vi "Get-client-channels-by-type.vi"(8 "error in (no error)":errorcluster, 10 "Module type":T1, 11 "ModComm in":T2) -> (0 "error out":errorcluster, 2 "Client channels":refnum<queue>[](array[refnum]), 3 "ModComm out":T2)   [LabVIEW 2013, in "Server.lvlib" / "Server.lvclass"]
uses:
  Server.lvclass
  Object-reference.ctl
  Supported-module-types.ctl
  Messages/Sources/Message.lvclass
  Server.lvclass/Server.ctl
  Read Clients.vi
  Read Client channels.vi
  Read Server channel.vi
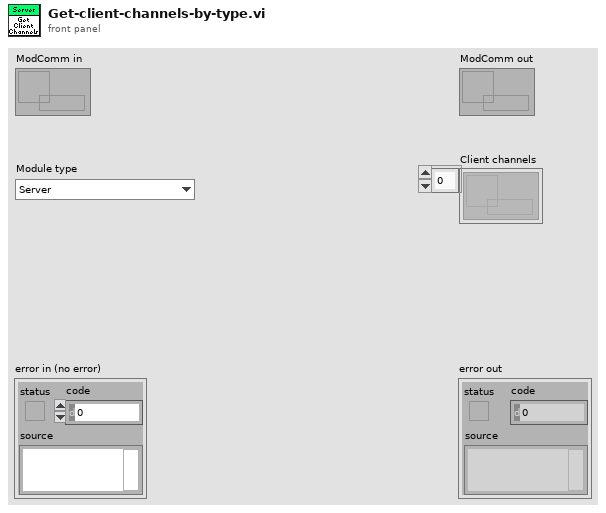
[diagram p1: front panel]
types:
  T1 = typedef "Server.lvlib/Server.lvclass/Supported-module-types.ctl" = enum16{"Server", "All", "BeamControl", "PowderDeposition", "StrategyParser", "CameraVision", "MaterialCharacterization", "StatusMonitor", "SLMSimulation", "LaserCharacterization"}
  T2 = typedef "Server.lvlib/Server.lvclass/Object-reference.ctl" = refnum<data-value>
  T3 = typedef "Module-communication.lvlib/Server.lvclass/Supported-module-types.ctl" = enum16{"Server", "All", "BeamControl", "PowderDeposition", "StrategyParser", "CameraVision", "MaterialCharacterization", "StatusMonitor", "SLMSimulation", "LaserCharacterization"}
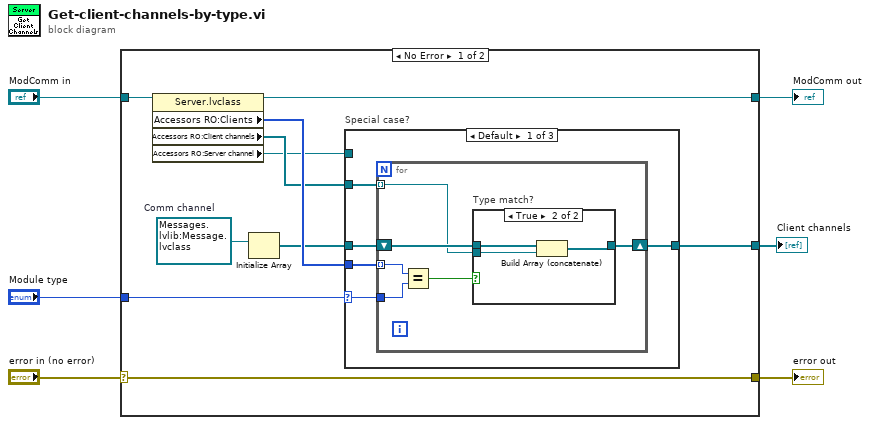
[diagram p0: block diagram]
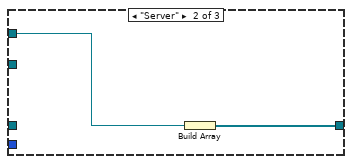
[diagram p3: hidden frame]
diagram:
  n1 = case shown="No Error" "error in (no error)" {
    selector: "error in (no error)" -> [w16 w36]
    tunnel: [w16 w36] -> w5
    tunnel: [w14 w35] -> w3
    tunnel: "ModComm in" -> [w15 w35]
    tunnel: "Module type" -> [w7 _]
    tunnel: [w12 _] -> w1
    frame No Error {
      w10 = refnum<queue> refnum  # Comm channel
      n2 = property class="Server.lvclass"(reference=w15) -> (reference out=w14:T2, "Accessors RO:Clients"=w13:T3[], "Accessors RO:Client channels"=w9:refnum<queue>[], "Accessors RO:Server channel"=w8:refnum<queue>)  [unwired: 1 in, 1 out]
      n3 = Initialize Array(w10) -> (w11:refnum<queue>[])  [unwired: 1 in]
      n4 = case "Special case?" shown="Default" w7 {
        selector: w7 -> [w17 _ _]
        tunnel: w13 -> [w21 _ _]
        tunnel: [w20 w32 w34] -> w12
        tunnel: w11 -> [w19 _ _]
        tunnel: w9 -> [w18 _ w34]
        tunnel: w8 -> [_ w33 _]
        frame Default {
          n5 = for {
            tunnel: w21 -> [w26] mode=indexing
            tunnel: w17 -> [w27]
            shift-right: [w22] -> w20
            shift-left: w19 -> [w25]
            tunnel: w18 -> [w23] mode=indexing
            n6 = Equal?(x=w26, y=w27) -> (x = y?=w24:bool)
            n7 = case "Type match?" shown="True" w24 {
              tunnel: w25 -> [w28 w31]
              tunnel: w23 -> [_ w30]
              tunnel: [w28 w29] -> w22
              frame False {
              }
              frame True {
                n8 = Build Array (concatenate)(w31, w30) -> (w29:refnum<queue>[])
              }
            }
          }
        }
        frame "Server" {
          n9 = Build Array(w33) -> (w32:refnum<queue>[])
        }
        frame "All" {
        }
      }
    }
    frame Error {
    }
  }
  "error out" <- w5
  "ModComm out" <- w3
  "Client channels" <- w1
